vi "FTDI - Read Unit.vi"(6 "Index":i32, 8 "error in":errorcluster, 11 "Result":u8[](array[numeric])=[2, 14, 34, 1, 0, 66, 62, 41, 121, 0, 0, 0, 0, 1]) -> (0 "error out":errorcluster, 2 "Data Unit":T1, 3 "Success":bool)   [LabVIEW 2019]
uses:
  Controls/Global - Unit.vi
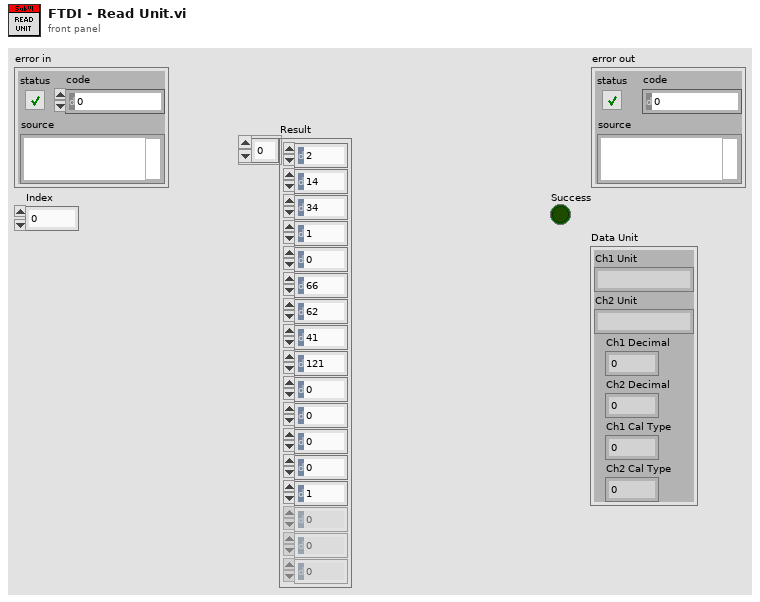
[diagram p1: front panel]
types:
  T1 = cluster{"Ch1 Unit":string, "Ch2 Unit":string, "Ch1 Decimal":u8, "Ch2 Decimal":u8, "Ch1 Cal Type":u8, "Ch2 Cal Type":u8}
  T2 = cluster{"Name":string[], "Unit":string[], "Decimal Point":u8[], "Ch Log":u8[], "H Alarm":u8[], "L Alarm":u8[], "H Limit":sgl[], "L Limit":sgl[], "Filter":u8[], "Gain":u8[], "Calib Type":u32[]}[]
  T3 = cluster{"Name":string[], "Unit":string[], "Decimal Point":u8[], "Ch Log":u8[], "H Alarm":u8[], "L Alarm":u8[], "H Limit":sgl[], "L Limit":sgl[], "Filter":u8[], "Gain":u8[], "Calib Type":u32[]}
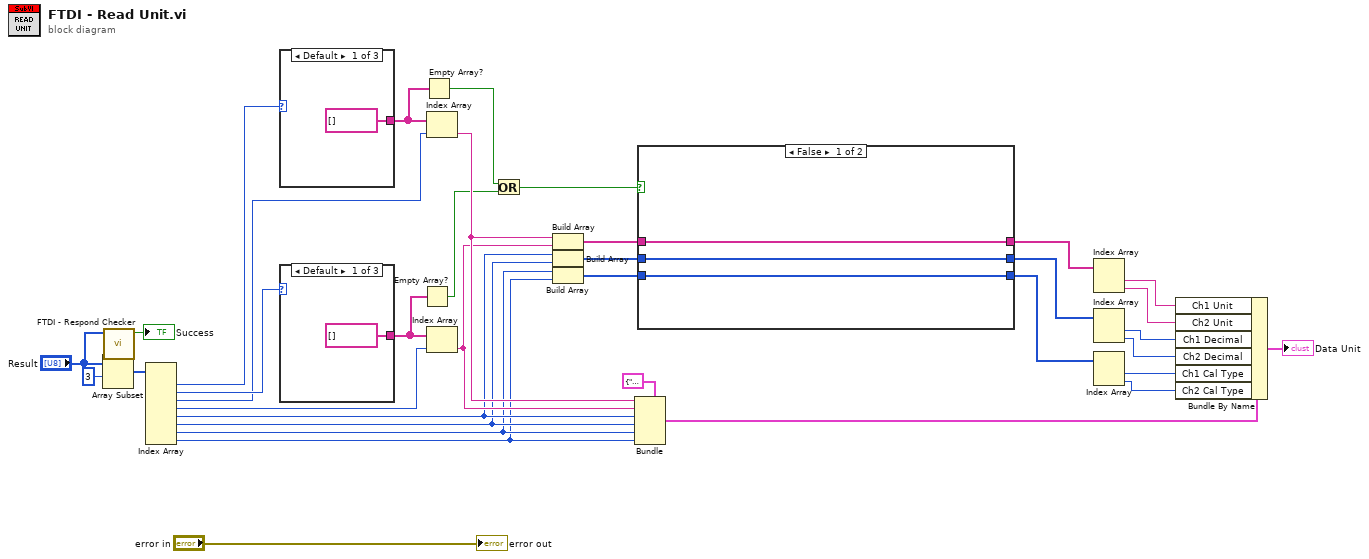
[diagram p0: block diagram]
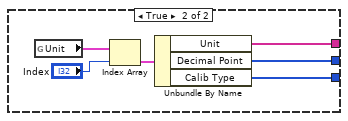
[diagram p2: hidden frame]
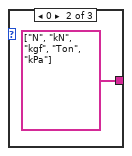
[diagram p3: hidden frame]
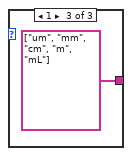
[diagram p4: hidden frame]
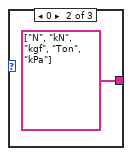
[diagram p5: hidden frame]
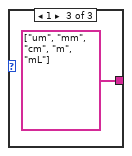
[diagram p6: hidden frame]
diagram:
  n1 = Array Subset(array="Result", index=3) -> (w34:u8[])  [unwired: 1 in]
  n2 = call "FTDI - Respond Checker.vi"("Read Data"="Result") -> ("Success"=→"Success":bool)  [unwired: 10 in]
  n3 = Index Array(array=w34) -> (element #1=w31:u8, element #2=w30:u8, element #3=w29:u8, element #4=w28:u8, element #5=w22:u8, element #6=w21:u8, element #7=w19:u8, element #8=w18:u8)  [unwired: 8 in]
  n4 = case shown="Default" w31 {
    tunnel: [string[] [] string[] ["N", "kN", "kgf", "Ton", "kPa"] string[] ["um", "mm", "cm", "m", "mL"]] -> w16
    frame Default {
    }
    frame 0 {
    }
    frame 1 {
    }
  }
  n5 = case shown="Default" w30 {
    tunnel: [string[] [] string[] ["N", "kN", "kgf", "Ton", "kPa"] string[] ["um", "mm", "cm", "m", "mL"]] -> w15
    frame Default {
    }
    frame 0 {
    }
    frame 1 {
    }
  }
  n6 = Empty Array?(array=w15) -> (empty?=w14:bool)
  n7 = Empty Array?(array=w16) -> (empty?=w13:bool)
  n8 = Index Array(array=w16, index=w29) -> (element=w25:string)
  n9 = Index Array(array=w15, index=w28) -> (element=w24:string)
  n10 = Or(x=w13, y=w14) -> (x .or. y?=w12:bool)
  n11 = Build Array(w25, w24) -> (w23:string[])
  n12 = Build Array(w22, w21) -> (w20:u8[])
  n13 = Build Array(w19, w18) -> (w17:u8[])
  n14 = Bundle(cluster=T1 {"Ch1 Unit"="", "Ch2 Unit"="", "Ch1 Decimal"=0, "Ch2 Decimal"=0, "Ch1 Cal Type"=0, "Ch2 Cal Type"=0}, "Ch1 Unit"=w25, "Ch2 Unit"=w24, "Ch1 Decimal"=w22, "Ch2 Decimal"=w21, "Ch1 Cal Type"=w19, "Ch2 Cal Type"=w18) -> (w11:T1)
  n15 = case shown="False" w12 {
    tunnel: w23 -> [w44 _]
    tunnel: w20 -> [w43 _]
    tunnel: w17 -> [w42 _]
    tunnel: [w44 w47] -> w3
    tunnel: [w43 w46] -> w2
    tunnel: [w42 w45] -> w1
    frame False {
    }
    frame True {
      n16 = global read "Global - Unit.vi" "Unit"() -> (w48:T2)
      n17 = Index Array(array=w48, index="Index") -> (element=w50:T3)
      n18 = Unbundle By Name(w50) -> ("Unit"=w47:string[], "Decimal Point"=w46:u8[], "Calib Type"=w45:u32[])
    }
  }
  n19 = Index Array(array=w3) -> (element #1=w9:string, element #2=w8:string)  [unwired: 2 in]
  n20 = Index Array(array=w2) -> (element #1=w7:u8, element #2=w6:u8)  [unwired: 2 in]
  n21 = Index Array(array=w1) -> (element #1=w5:u32, element #2=w4:u32)  [unwired: 2 in]
  n22 = Bundle By Name(cluster=w11, "Ch1 Unit"=w9, "Ch2 Unit"=w8, "Ch1 Decimal"=w7, "Ch2 Decimal"=w6, "Ch1 Cal Type"=w5, "Ch2 Cal Type"=w4) -> (→"Data Unit":T1)
  "error out" <- "error in"
